vi "Init Device.vi"(8 "error in (no error)":errorcluster, 11 "Device in":refnum<class "CK.lvclass">) -> (0 "error out":errorcluster, 3 "Device out":refnum<class "CK.lvclass">)   [LabVIEW 2020, in "CK.lvclass"]
doc: "Init the device com port.\nThis should be called by the child class and the child class is responsible for setting the device as its default state."
uses:
  CK.lvclass
  PIC-device/PIC-Device.lvclass
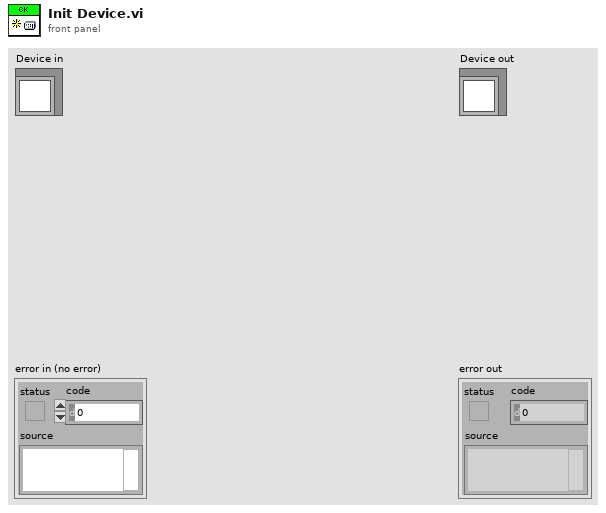
[diagram p1: front panel]
types:
  T1 = typedef "PIC-Device.lvclass/Register to Write.ctl" = cluster{"Register":u32, "Value":u32, "Dev Address":u32, "Physical Adress":u32}
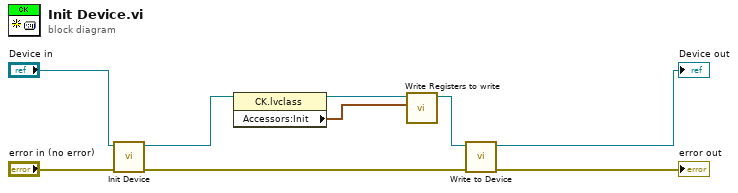
[diagram p0: block diagram]
diagram:
  n1 = call-parent "Init Device.vi"("error in (no error)"="error in (no error)", "Device in"="Device in") -> ("error out"=w2:errorcluster, "Device out"=w4:refnum<class "CK.lvclass">)  [unwired: 8 in]
  n2 = property class="CK.lvclass"(reference=w4) -> (reference out=w5:refnum<class "CK.lvclass">, "Accessors:Init"=w6:T1[])  [unwired: 1 in, 1 out]
  n3 = call-dynamic "Write Registers to write.vi"("Registers to write"=w6, "Device in"=w5) -> ("Device out"=w7:refnum<class "CK.lvclass">)  [unwired: 9 in]
  n4 = call-dynamic "Write to Device.vi"("error in (no error)"=w2, "Device in"=w7) -> ("error out"=→"error out":errorcluster, "Device out"=→"Device out":refnum<class "CK.lvclass">)  [unwired: 7 in, 1 out]
